vi "Chrg_Dschrg_No_cDAQ2.vi"(0 "file path (use dialog)":path, 4 "PS VISA in":refnum<visa-resource-name>, 5 "PS error in":errorcluster, 6 "DischargeCyclePath":path=path "C:/Users/ga11/Desktop/VI/results/3PtestCharge.lvm" caption="Filename", 8 "Charge/discharge":enum8{"Charge", "Discharge"}(ring), 9 "Charge/Discharge Voltage Setpoint":dbl format="%#.6g", 10 "CC or CCCV":enum16{"CC", "CCCV"}(ring), 11 "Current Setpoint":dbl format="%#.6g", 12 "Output Safety":T1, 13 "Current Cutoff":dbl) -> (18 "PS VIS resource name out":refnum<visa-resource-name>, 19 "PS error out":errorcluster)   [LabVIEW 2020]
uses:
  Drivers-NHR-9200/NHR/Public/Data/Low Level/Fetch (Ave Voltage).vi
  Control-Applications/Global_Stop_3.vi
  Drivers-NHR-9200/NHR/NH Research Regenerative Test Series.lvlib
panel:
  out "Read Ave Current (A)":dbl
  out "Read Ave Voltage (V)":dbl
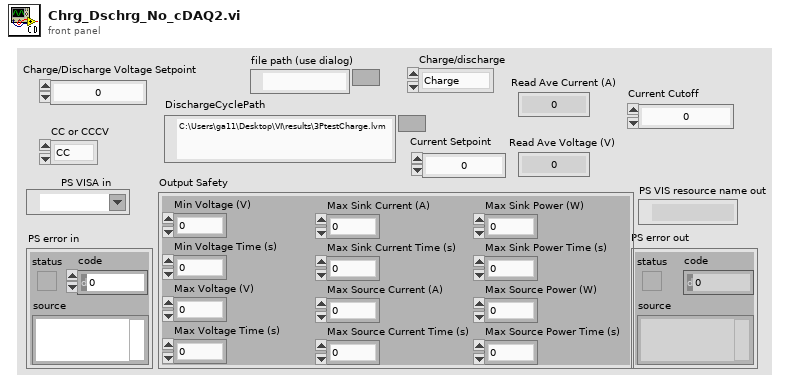
[diagram p1: front panel]
types:
  T1 = cluster{"Min Voltage (V)":dbl, "Min Voltage Time (s)":dbl, "Max Voltage (V)":dbl, "Max Voltage Time (s)":dbl, "Max Sink Current (A)":dbl, "Max Sink Current Time (s)":dbl, "Max Source Current (A)":dbl, "Max Source Current Time (s)":dbl, "Max Sink Power (W)":dbl, "Max Sink Power Time (s)":dbl, "Max Source Power (W)":dbl, "Max Source Power Time (s)":dbl}
  T2 = enum16{"open", "replace", "create", "open or create", "replace or create", "replace or create with confirmation"}
  T3 = cluster{"Voltage Enabled":bool, "Current Enabled":bool, "Power Enabled":bool, "Resistance Enabled":bool}
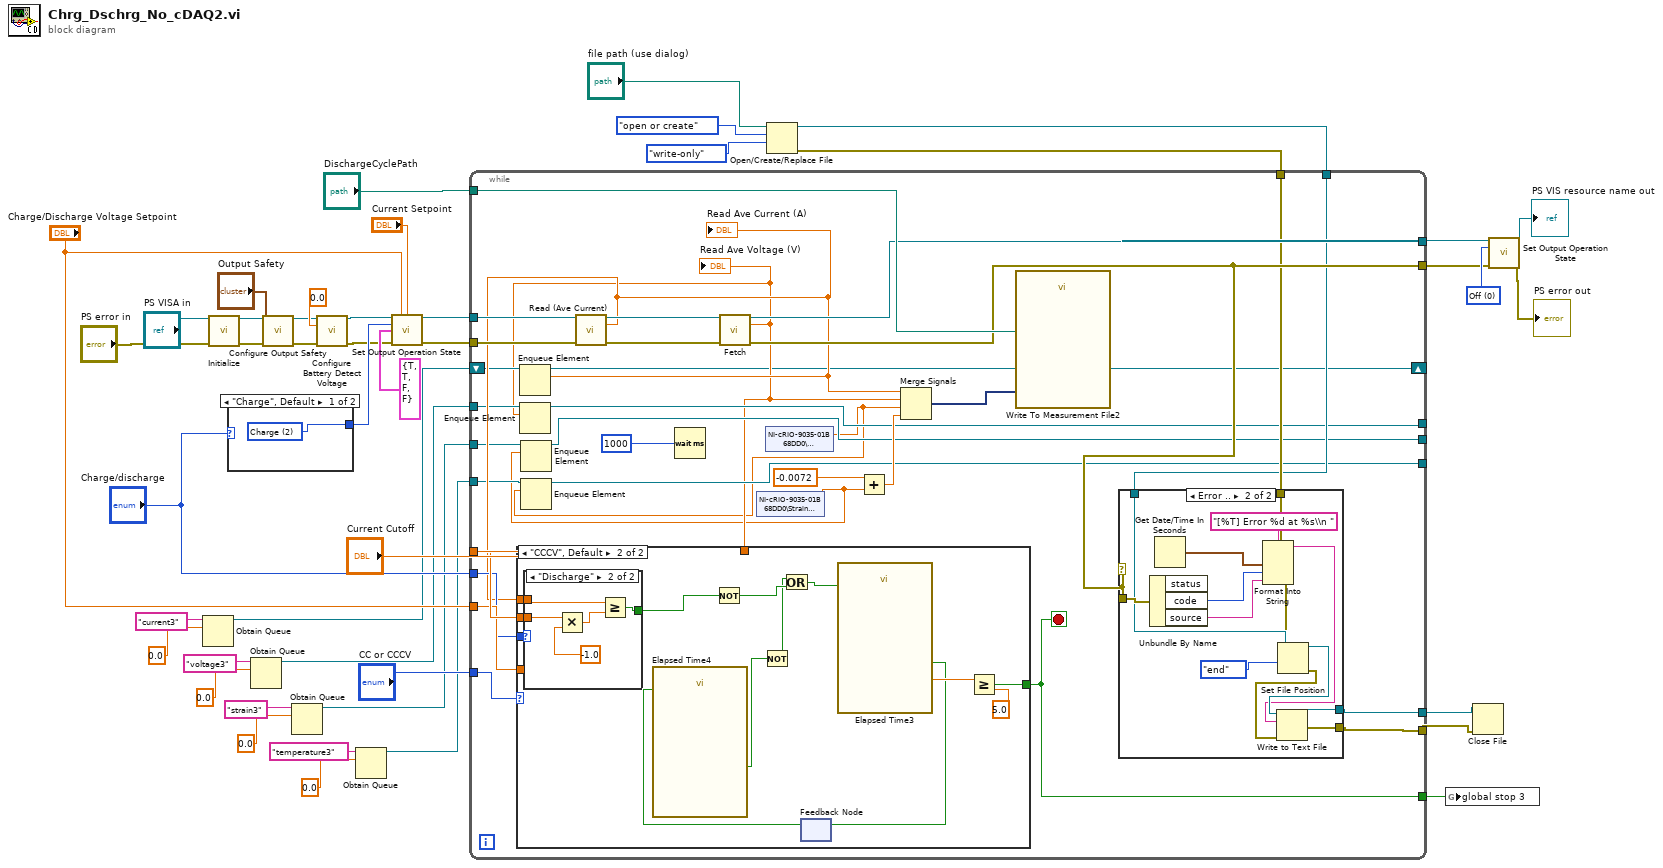
[diagram p0: block diagram]
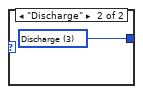
[diagram p2: hidden frame]
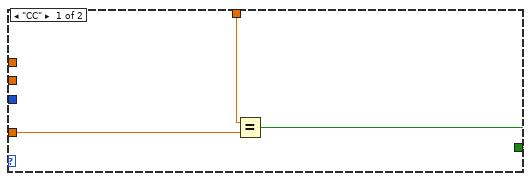
[diagram p4: hidden frame]
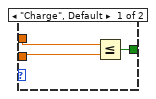
[diagram p5: hidden frame]
diagram:
  w34 = 0 items=["Off", "Standby", "Charge", "Discharge", "Battery"] ("Mode (0: Off)")
  n1 = Obtain Queue(name (unnamed)="current3", element data type=0.0) -> (queue out=w4:refnum<queue>)  [unwired: 3 in, 2 out]
  n2 = call "Initialize.vi"("VISA resource name"="PS VISA in", "error in (no error)"="PS error in") -> ("VISA resource name out"=w25:refnum<visa-resource-name>, "error out"=w26:errorcluster)  [unwired: 12 in]
  n3 = case shown="\"Charge\", Default" "Charge/discharge" {
    tunnel: [w46 w47] -> w35
    frame "Charge", Default {
      w46 = 2 items=["Off", "Standby", "Charge", "Discharge", "Battery"] ("Mode (0: Off)")
    }
    frame "Discharge" {
      w47 = 3 items=["Off", "Standby", "Charge", "Discharge", "Battery"] ("Mode (0: Off)")
    }
  }
  n4 = Obtain Queue(name (unnamed)="voltage3", element data type=0.0) -> (queue out=w3:refnum<queue>)  [unwired: 3 in, 2 out]
  n5 = call "Configure Output Safety.vi"("VISA resource name"=w25, "Output Safety"="Output Safety", "error in (no error)"=w26) -> ("VISA resource name out"=w28:refnum<visa-resource-name>, "error out"=w27:errorcluster)  [unwired: 11 in]
  n6 = Obtain Queue(name (unnamed)="strain3", element data type=0.0) -> (queue out=w2:refnum<queue>)  [unwired: 3 in, 2 out]
  n7 = call "Configure Battery Detect Voltage.vi"("VISA resource name"=w28, "Battery Detect Voltage (0V)"=0.0, "error in (no error)"=w27) -> ("VISA resource name out"=w33:refnum<visa-resource-name>, "error out"=w32:errorcluster)  [unwired: 11 in]
  n8 = Obtain Queue(name (unnamed)="temperature3", element data type=0.0) -> (queue out=w1:refnum<queue>)  [unwired: 3 in, 2 out]
  n9 = call "Set Output Operation State.vi"("VISA resource name"=w33, "Voltage Setpoint (0 V)"="Charge/Discharge Voltage Setpoint", "Current Setpoint (0 A)"="Current Setpoint", "Mode (0: Off)"=w35, "Enable"=T3 {"Voltage Enabled"=TRUE, "Current Enabled"=TRUE, "Power Enabled"=FALSE, "Resistance Enabled"=FALSE}, "error in (no error)"=w32) -> ("VISA resource name out"=w38:refnum<visa-resource-name>, "error out"=w37:errorcluster)  [unwired: 8 in]
  n10 = Open/Create/Replace File(file path (use dialog)="file path (use dialog)", operation (0:open)=T2."open or create", access (0:read/write)=enum16{"read/write", "read-only", "write-only"}."write-only") -> (refnum out=w14:refnum<file>, error out=w15:errorcluster)  [unwired: 3 in, 1 out]
  n11 = while {
    tunnel: w38 -> [w77]
    tunnel: w37 -> [w76]
    tunnel: "Current Cutoff" -> [w71]
    tunnel: "DischargeCyclePath" -> [w73]
    tunnel: [w72] -> w30
    tunnel: [w63] -> w29
    tunnel: "CC or CCCV" -> [w70]
    tunnel: "Charge/Discharge Voltage Setpoint" -> [w69]
    tunnel: "Charge/discharge" -> [w68]
    tunnel: [w65] -> w20
    tunnel: [w64] -> w19
    tunnel: w15 -> [w62]
    tunnel: w14 -> [w61]
    shift-right: [w48] -> _
    shift-left: w4 -> [w58]
    tunnel: [w60] -> w11
    tunnel: w3 -> [w57]
    tunnel: w2 -> [w56]
    tunnel: w1 -> [w55]
    tunnel: [w54] -> _
    tunnel: [w53] -> _
    tunnel: [w52] -> _
    stop <- w60 stop-if-true
    n12 = call "Read (Ave Current).vi"("VISA resource name"=w77, "error in (no error)"=w76) -> ("VISA resource name out"=w78:refnum<visa-resource-name>, "Ave Current (A)"=w59:dbl, "error out"=w79:errorcluster)  [unwired: 11 in]
    "Read Ave Current (A)" <- w59
    n13 = Enqueue Element(queue=w58, element=w59) -> (queue out=w48:refnum<queue>)  [unwired: 2 in, 2 out]
    n14 = Wait (ms)(milliseconds to wait=1000) -> ()  [unwired: 1 out]
    n15 = call-poly "Fetch.vi"("VISA resource name"=w78, "error in (no error)"=w79) -> ("VISA resource name out"=w72:refnum<visa-resource-name>, "Ave Voltage (V)"=w51:dbl, "error out"=w63:errorcluster)  [unwired: 11 in]
    "Read Ave Voltage (V)" <- w51
    n16 = case shown="\"CCCV\", Default" w70 {
      tunnel: [w96 w105] -> w60
      tunnel: w71 -> [_ w102]
      tunnel: w59 -> [_ w101]
      tunnel: w51 -> [w98 _]
      tunnel: w69 -> [w97 _]
      tunnel: w68 -> [_ w99]
      frame "CC" {
        n17 = Equal?(x=w98, y=w97) -> (x = y?=w96:bool)
      }
      frame "CCCV", Default {
        n18 = case shown="\"Discharge\"" w99 {
          tunnel: w102 -> [w113 w118]
          tunnel: w101 -> [w114 w116]
          tunnel: [w112 w115] -> w100
          frame "Charge", Default {
            n19 = Less Or Equal?(x=w114, y=w113) -> (x <= y?=w112:bool)
          }
          frame "Discharge" {
            n20 = Multiply(x=w118, y=-1.0) -> (x*y=w117:dbl)
            n21 = Greater Or Equal?(x=w116, y=w117) -> (x >= y?=w115:bool)
          }
        }
        n22 = Not(x=w100) -> (.not. x?=w111:bool)
        n23 = feedback #1() -> (w103:bool)  [unwired: 1 in]
        n24 = call "Elapsed Time4"("Reset"=w103) -> ("Time has Elapsed"=w110:bool)  [unwired: 11 in, 7 out]
        n25 = Not(x=w110) -> (.not. x?=w109:bool)
        n26 = Or(x=w109, y=w111) -> (x .or. y?=w108:bool)
        n27 = call "Elapsed Time3"("Reset"=w108) -> ("Elapsed Time (s)"=w107:dbl, "Time has Elapsed"=w104:bool)  [unwired: 11 in, 6 out]
        n28 = feedback-in #1(w104) -> ()
        n29 = Greater Or Equal?(x=w107, y=5.0) -> (x >= y?=w105:bool)
      }
    }
    n30 = Enqueue Element(queue=w57, element=w51) -> (queue out=w52:refnum<queue>)  [unwired: 2 in, 2 out]
    n31 = shared-variable "NI-cRIO-9035-01B68DD0\\Strain Gauge\\SGI2"() -> (w50:dbl)  [unwired: 1 in, 1 out]
    n32 = Enqueue Element(queue=w56, element=w50) -> (queue out=w53:refnum<queue>)  [unwired: 2 in, 2 out]
    n33 = shared-variable "NI-cRIO-9035-01B68DD0\\Thermocouple\\TCI2"() -> (w49:dbl)  [unwired: 1 in, 1 out]
    n34 = Enqueue Element(queue=w55, element=w49) -> (queue out=w54:refnum<queue>)  [unwired: 2 in, 2 out]
    n35 = Add(x=-0.0072, y=w50) -> (x+y=w66:dbl)
    n36 = Merge Signals "Merge Signals"(w59, w51, w49, w66) -> (w75:dynamicdata)
    n37 = call "Write To Measurement File2"("Signals"=w75, "Filename"=w73) -> ()  [unwired: 15 in, 3 out]
    n38 = case shown="Error .." w63 {
      tunnel: w63 -> [_ w95]
      tunnel: w61 -> [w81 w93]
      tunnel: [w81 w91] -> w65
      tunnel: w62 -> [w80 w90]
      tunnel: [w80 w87] -> w64
      frame No Error {
      }
      frame Error {
        n39 = Unbundle By Name(w95) -> ("code"=w84:i32, "source"=w83:string)  [unwired: 1 out]
        n40 = Get Date/Time In Seconds() -> (seconds since 1Jan1904=w85:timestamp)
        n41 = Format Into String(format string="[%T] Error %d at %s\\n ", error in=w90, w85, w84, w83) -> (resulting string=w82:string, error out=w89:errorcluster)  [unwired: 1 in]
        n42 = Set File Position(refnum=w93, from (0:start)=enum16{"start", "end", "current"}."end", error in=w89) -> (refnum out=w92:refnum<file>, error out=w88:errorcluster)  [unwired: 1 in]
        n43 = Write to Text File(file (use dialog)=w92, text=w82, error in=w88) -> (refnum out=w91:refnum<file>, error out=w87:errorcluster)  [unwired: 1 in, 1 out]
      }
    }
  }
  n44 = global write "Global_Stop_3.vi" "global stop 3"(w11) -> ()
  n45 = Close File(refnum=w20, error in=w19) -> ()  [unwired: 2 out]
  n46 = call "Set Output Operation State.vi"("VISA resource name"=w30, "Mode (0: Off)"=w34, "error in (no error)"=w29) -> ("VISA resource name out"=→"PS VIS resource name out":refnum<visa-resource-name>, "error out"=→"PS error out":errorcluster)  [unwired: 11 in]
